vi "Gauge_tb.vi"() -> ()   [LabVIEW 2018]
uses:
  <instrlib>/MKS 972B/Public/Utility/Unit address.ctl
  <instrlib>/MKS 972B/MKS 972B.lvlib
panel:
  in  "stop":bool
  in  "Pressure unit":string(combo)="mbar"
  in  "Calibration gas type":string(combo)="AIR"
  out "chart":dbl(graph)
  out "Pressure value":dbl
  in  "Reading mode":u16(ring)=1 items=["MicroPirani value (3 digits)"=1, "Cold Cathode value (3 digits)"=2, "Combined (3 digits)"=3, "Combined (4 digits)"=4]
  in  "Unit address":T1=1 min=1 max=255 format="%03d"
  in  "VISA resource name":refnum<visa-resource-name>="COM1"
  in  "Serial Configuration":T2={"Baud Rate"=9600, "Parity"=0, "Data Bits"=8, "Stop Bits"=10, "Flow Control"=0} {"Flow Control" items=["None", "XON/XOFF", "RTS/CTS", "XON/XOFF & RTS/CTS", "DTR/DSR", "XON/XOFF & DTR/DSR"]; "Stop Bits" items=["1.0"=10, "1.5"=15, "2.0"=20]; "Data Bits" items=["7"=7, "8"=8]; "Parity" items=["None", "Odd", "Even", "Mark", "Space"]; "Baud Rate" items=["300"=300, "600"=600, "1200"=1200, "2400"=2400, "4800"=4800, "9600"=9600, "19200"=19200]}
  # "This program is an standalong version that\noperates the vacuum gauge. The program\nfirst initialize the gauge with baud rate, reading\nmode and unit address.  It than set the calibration\ngas type and the pressue unit.  After that, the \nprogram enters an inifite loop that continusouly\nread the current value and plot them out..\nWhenever the user press the stop button, the \nprogram stops reading and execute final commend\nto turnoff the sensor."
  # "The unit address is what address the gauge is \nallocated in RS485. By default, we use 253 according to \nthe manual. However, the final unit address might\nbe different since there are lots of instrument\nconnected together and each instrument MUST\nhave a UNIQUE unit address.\nThe unit address, used for serail communication, \n ranges from 1 to 255."
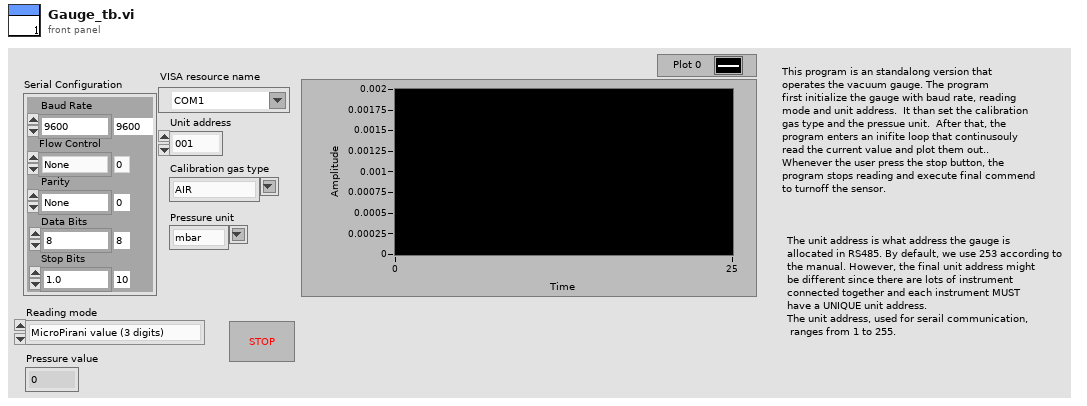
[diagram p1: front panel]
types:
  T1 = typedef "MKS 972B.lvlib/Unit address.ctl" = u32
  T2 = cluster{"Baud Rate":u32, "Parity":u16, "Data Bits":u16, "Stop Bits":u16, "Flow Control":u16}
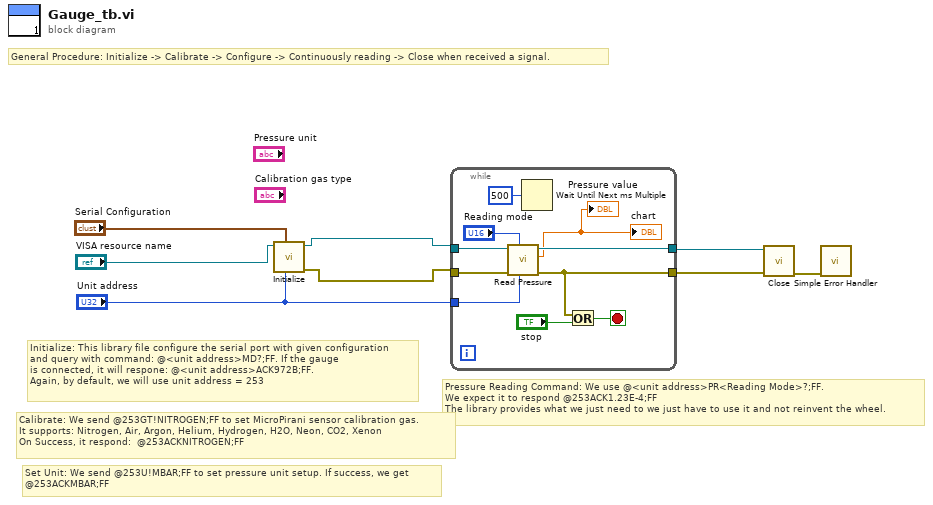
[diagram p0: block diagram]
diagram:
  # "Set Unit: We send @253U!MBAR;FF to set pressure unit setup. If success, we get\n@253ACKMBAR;FF"
  # "Calibrate: We send @253GT!NITROGEN;FF to set MicroPirani sensor calibration gas.\nIt supports: Nitrogen, Air, Argon, Helium, Hydrogen, H2O, Neon, CO2, Xenon\nOn Success, it respond:  @253ACKNITROGEN;FF"
  # "Initialize: This library file configure the serial port with given configuration\nand query with command: @<unit address>MD?;FF. If the gauge\nis connected, it will respone: @<unit address>ACK972B;FF. \nAgain, by default, we will use unit address = 253"
  # "Pressure Reading Command: We use @<unit address>PR<Reading Mode>?;FF. \nWe expect it to respond @253ACK1.23E-4;FF\nThe library provides what we just need to we just have to use it and not reinvent the wheel."
  # "General Procedure: Initialize -> Calibrate -> Configure -> Continuously reading -> Close when received a signal."
  n1 = call <instrlib>:"Initialize.vi"("Unit address to query ID (001-254)"="Unit address", "Serial Configuration"="Serial Configuration", "VISA resource name"="VISA resource name") -> ("error out"=w1:errorcluster, "VISA resource name out"=w2:refnum<visa-resource-name>)  [unwired: 7 in]
  n2 = while {
    tunnel: w1 -> [w17]
    tunnel: w2 -> [w16]
    tunnel: [w15] -> w4
    tunnel: [w13] -> w3
    tunnel: "Unit address" -> [w12]
    stop <- w14 stop-if-true
    n3 = call <instrlib>:"Read Pressure.vi"("Unit address (001-253)"=w12, "Reading mode"="Reading mode", "error in (no error)"=w17, "VISA resource name"=w16) -> ("error out"=w13:errorcluster, "Pressure value"=→"Pressure value" →"chart":dbl, "VISA resource name out"=w15:refnum<visa-resource-name>)  [unwired: 5 in]
    n4 = Wait Until Next ms Multiple(millisecond multiple=u32 500) -> ()  [unwired: 1 out]
    n5 = Or(x=w13, y="stop") -> (x .or. y?=w14:bool)
  }
  n6 = call <instrlib>:"Close.vi"("error in (no error)"=w3, "VISA resource name"=w4) -> ("error out"=w5:errorcluster)  [unwired: 9 in]
  n7 = call <vilib>:"Simple Error Handler.vi"("error in (no error)"=w5) -> ()  [unwired: 4 in, 5 out]
